vi "Filter Optional Data Replay Ctls.vi"(7 "Replay#":string, 10 "Numbers":string[](array[string]), 11 "Found in":bool[](array[boolean])) -> (3 "Found out":bool[](array[boolean]))   [LabVIEW 2011, in "Engine Sim System Explorer.lvlib"]
uses:
  Engine Sim System Explorer.lvlib
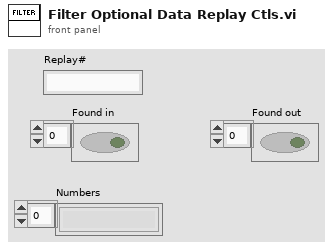
[diagram p1: front panel]
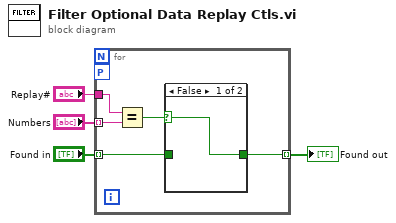
[diagram p0: block diagram]
diagram:
  n1 = for {
    tunnel: "Found in" -> [w5] mode=indexing
    tunnel: "Numbers" -> [w9] mode=indexing
    tunnel: "Replay#" -> [w8]
    tunnel: [w6] -> w1 mode=indexing
    workers-P: _ -> [_]
    n2 = Equal?(x=w8, y=w9) -> (x = y?=w7:bool)
    n3 = case shown="False" w7 {
      selector: w7 -> [w10 _]
      tunnel: [w10 w11] -> w6
      tunnel: w5 -> [_ w11]
      frame False {
      }
      frame True {
      }
    }
  }
  "Found out" <- w1
